vi "tsapp_add_cyclic_msg_can.vi"(8 "错误输入（无错误）":errorcluster, 9 "APeriodMS":sgl, 10 "TCAN":T1 {"AIsData" items=["Data Frame", "Remote Frame"]; "AIsStd" items=["Standard Frame", "Extended Frame"]; "AId" format="%x"; "AIdxchn" items=["CHN1", "CHN2", "CHN3", "CHN4", "CHN5", "CHN6", "CHN7", "CHN8", "CHN9", "CHN10", "CHN11", "CHN12", "CHN13", "CHN14", "CHN15", "CHN16", "CHN17", "CHN18", "CHN19", "CHN20", "CHN21", "CHN22", "CHN23", "CHN24", "CHN25", "CHN26", "CHN27", "CHN28", "CHN29", "CHN30", "CHN31", "CHN32"]}, 11 "path":path) -> (0 "错误输出":errorcluster, 2 "return":i32, 3 "path out":path)   [LabVIEW 2014]
doc: "Function Introduction :\nAfter adding periodic messages, TsMasterApi automatically completes the periodic sending of messages.\nCall location :\nIn situations where periodic transmission of CAN messages is required\ninput parameter :\nACAN: CAN message data\nAPeriodMS: Cycle value\nReturn value :\n==0: Added successfully\nOther values: Add failed, query error code"
uses:
  Typedef/TLibCAN.ctl
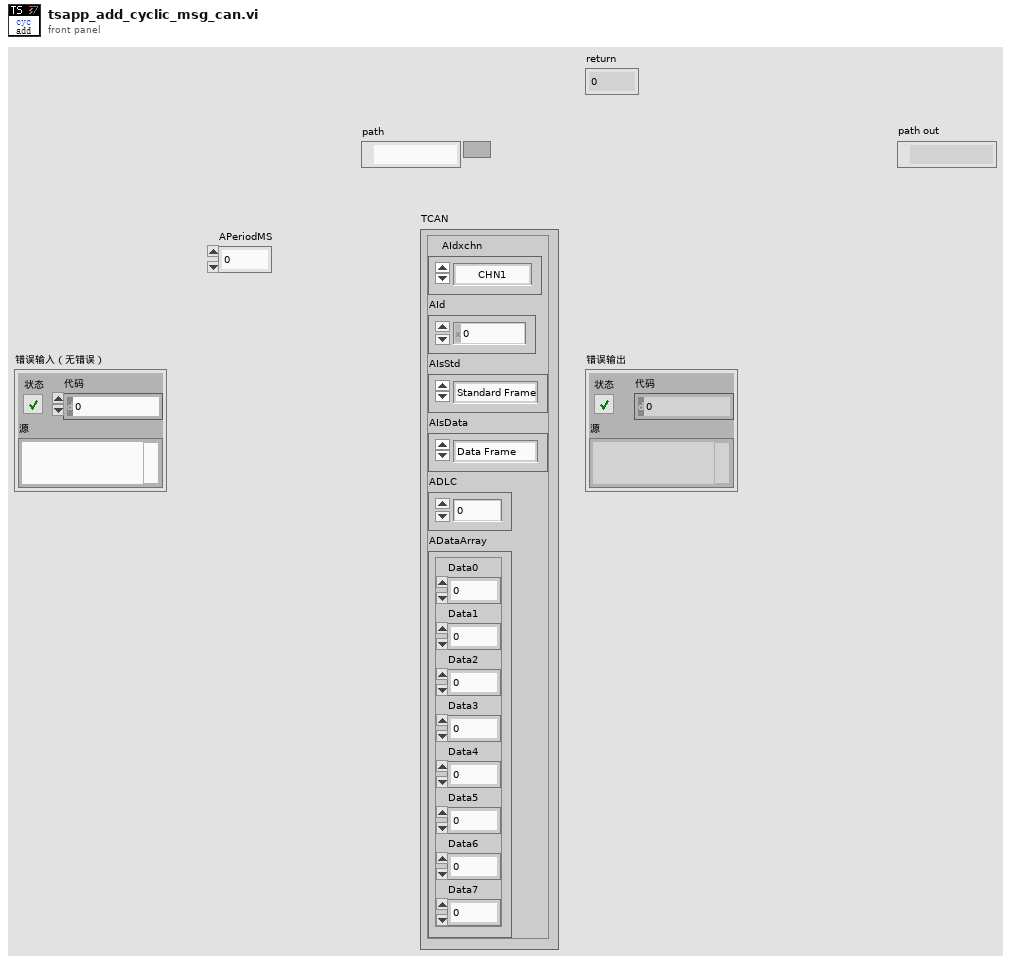
[diagram p1: front panel]
types:
  T1 = typedef "TLibCAN.ctl" = cluster{"AIdxchn":u8, "AId":i32, "AIsStd":u8, "AIsData":u8, "ADLC":u8, "ADataArray":cluster{"Data0":u8, "Data1":u8, "Data2":u8, "Data3":u8, "Data4":u8, "Data5":u8, "Data6":u8, "Data7":u8}}
  T2 = cluster{"FIdxChn":u8, "FProperties":u8, "FDLC":u8, "FReserved":u8, "FIdentifier":i32, "FTimeUS":u64, "Data0":u8, "Data1":u8, "Data2":u8, "Data3":u8, "Data4":u8, "Data5":u8, "Data6":u8, "Data7":u8}
  T3 = cluster{"FIdxChn":u8, "FProperties":u8, "FDLC":u8, "FReserved":u8, "FIdentifier":i32, "FTimeUS":u64, "FData":cluster{"Data0":u8, "Data1":u8, "Data2":u8, "Data3":u8, "Data4":u8, "Data5":u8, "Data6":u8, "Data7":u8}}
  T4 = cluster{"istx":bool, "remoteframe":bool, "extframe":bool, "tbd1":bool, "tbd2":bool, "tbd3":bool, "tbd4":bool, "iserrorframe":bool}
  T5 = cluster{"Data0":u8, "Data1":u8, "Data2":u8, "Data3":u8, "Data4":u8, "Data5":u8, "Data6":u8, "Data7":u8}
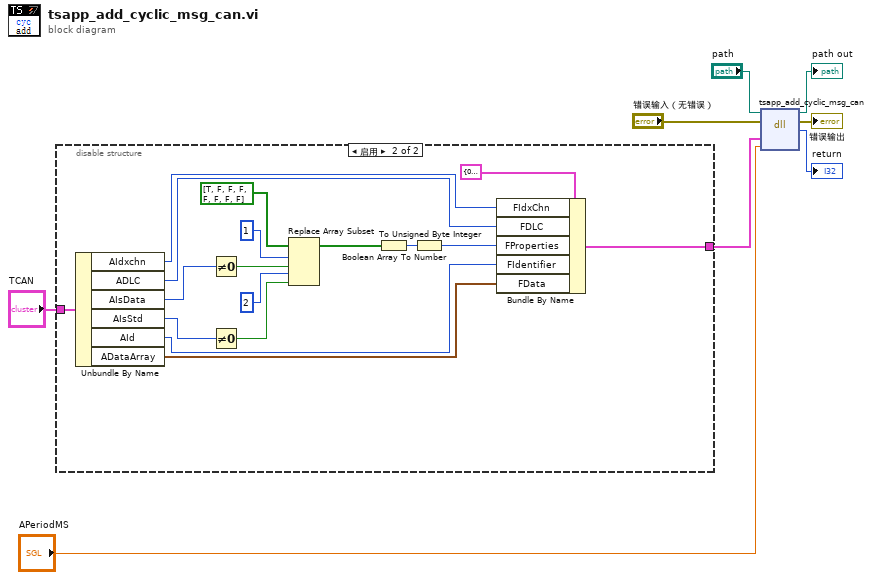
[diagram p0: block diagram]
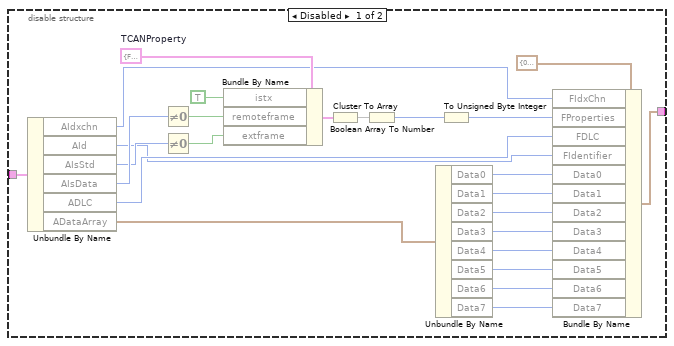
[diagram p2: hidden frame]
diagram:
  n1 = disable-structure shown="启用" {
    disable-tunnel: [w24 w34] -> w6
    disable-tunnel: "TCAN" -> [w23 w35]
    frame Disabled {
      w32 = T4 {"istx"=FALSE, "remoteframe"=FALSE, "extframe"=FALSE, "tbd1"=FALSE, "tbd2"=FALSE, "tbd3"=FALSE, "tbd4"=FALSE, "iserrorframe"=FALSE}  # TCANProperty
      n2 = Unbundle By Name(w23) -> ("AIdxchn"=w22:u8, "AId"=w18:i32, "AIsStd"=w20:u8, "AIsData"=w21:u8, "ADLC"=w19:u8, "ADataArray"=w17:T5)
      n3 = Not Equal To 0?(x=w21) -> (x != 0?=w26:bool)
      n4 = Not Equal To 0?(x=w20) -> (x != 0?=w25:bool)
      n5 = Bundle By Name(cluster=w32, "istx"=TRUE, "remoteframe"=w26, "extframe"=w25) -> (w28:T4)
      n6 = Cluster To Array(cluster=w28) -> (array=w30:bool[])
      n7 = Boolean Array To Number(Boolean array=w30) -> (number=w29:u32)
      n8 = Unbundle By Name(w17) -> ("Data0"=w16:u8, "Data1"=w15:u8, "Data2"=w14:u8, "Data3"=w13:u8, "Data4"=w12:u8, "Data5"=w11:u8, "Data6"=w10:u8, "Data7"=w9:u8)
      n9 = To Unsigned Byte Integer(number=w29) -> (unsigned 8bit integer=w27:u8)
      n10 = Bundle By Name(cluster=T2 {"FIdxChn"=0, "FProperties"=0, "FDLC"=0, "FReserved"=0, "FIdentifier"=0, "FTimeUS"=0, "Data0"=0, "Data1"=0, "Data2"=0, "Data3"=0, "Data4"=0, "Data5"=0, "Data6"=0, "Data7"=0} ("SendMsgInfo"), "FIdxChn"=w22, "FProperties"=w27, "FDLC"=w19, "FIdentifier"=w18, "Data0"=w16, "Data1"=w15, "Data2"=w14, "Data3"=w13, "Data4"=w12, "Data5"=w11, "Data6"=w10, "Data7"=w9) -> (w24:T2)
    }
    frame Enabled {
      n11 = Unbundle By Name(w35) -> ("AIdxchn"=w47:u8, "ADLC"=w37:u8, "AIsData"=w46:u8, "AIsStd"=w45:u8, "AId"=w48:i32, "ADataArray"=w49:T5)
      n12 = Not Equal To 0?(x=w46) -> (x != 0?=w42:bool)
      n13 = Not Equal To 0?(x=w45) -> (x != 0?=w40:bool)
      n14 = Replace Array Subset(array=bool[] [TRUE, FALSE, FALSE, FALSE, FALSE, FALSE, FALSE, FALSE], new element #1=w42, index #1=1 ("索引"), new element #2=w40, index #2=2 ("索引")) -> (w39:bool[])
      n15 = Boolean Array To Number(Boolean array=w39) -> (number=w38:u32)
      n16 = To Unsigned Byte Integer(number=w38) -> (unsigned 8bit integer=w36:u8)
      n17 = Bundle By Name(cluster=T3 {"FIdxChn"=0, "FProperties"=0, "FDLC"=0, "FReserved"=0, "FIdentifier"=0, "FTimeUS"=0, "FData"={"Data0"=0, "Data1"=0, "Data2"=0, "Data3"=0, "Data4"=0, "Data5"=0, "Data6"=0, "Data7"=0}} ("簇"), "FIdxChn"=w47, "FDLC"=w37, "FProperties"=w36, "FIdentifier"=w48, "FData"=w49) -> (w34:T3)
    }
  }
  n18 = dll-call lib="PTH2Zabs CUsers\nAdministratorDesktop海卓电堆系统程序\nTS_CAN_ModTSMaster.dll" fn="tsapp_add_cyclic_msg_can"(path in="path", error in="错误输入（无错误）", "ACAN"=w6, "Cyclie"="APeriodMS") -> (path out=→"path out":path, error out=→"错误输出":errorcluster, "tsapp_add_cyclic_msg_can"=→"return":i32)  [unwired: 3 in]
